vi "updateWaypoints.vi"(8 "error in (no error)":errorcluster, 11 "StationKeeping in":refnum<class "StationKeeping.lvclass">) -> (0 "error out":errorcluster, 3 "StationKeeping out":refnum<class "StationKeeping.lvclass">)   [LabVIEW 2011, in "StationKeeping.lvclass"]
doc: "Handles the 3 phases of the station keeping mission, while it is in progress. First, it checks if the mission should be started, by checking if the robot is in the station or not. If not, the start time is reset for the mission.\nIf so, using a timer, it checks which phase of the mission it is in. In the first phase, it calls \"station_keeping_waypoints.vi\" and adds waypoints to the waypoints array from a pattern in that VI. In the second phase, it adds waypoints along the edge of the boundary. These are 7 meters from the corners regardless of station size. In the third phase, it adds a waypoint outside the boundary (w/out a No-Sail Zone)\n\nThe purpose of the Local Variable \"Phase\" is to check when the phase is changing. The first time a phase changes, the \"current waypoint\" global is updated, in order to check off unecessary waypoints."
uses:
  StationKeeping.lvclass
  StationKeeping.lvclass/StationKeeping.ctl
  2 Globals/2 Global.vi
  Waypoint/Waypoint.lvclass
panel:
  out "Phase":dbl
  out "Time Elapsed":dbl
  out "Time Remaining":dbl
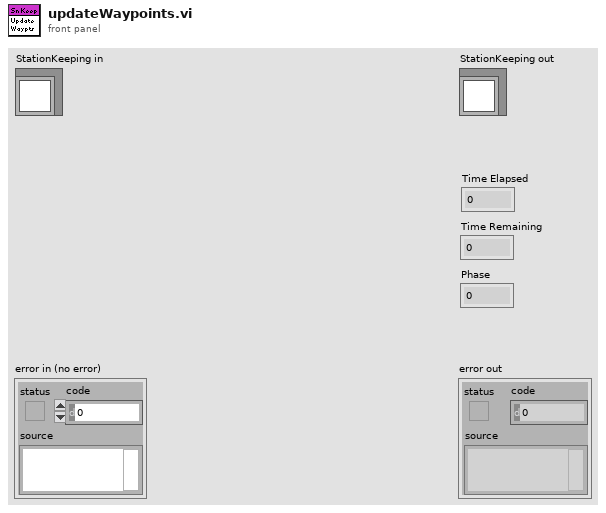
[diagram p1: front panel]
types:
  T1 = typedef "UTM Location.ctl" = cluster{"UTM Zone":dbl, "Hemisphere":enum16{"North", "South"}, "East":dbl, "North":dbl}
  T2 = typedef "UTM Circle.ctl" = cluster{"UTM Zone":dbl, "Hemisphere":enum16{"North", "South"}, "East":dbl, "North":dbl, "Radius":dbl}
  T3 = typedef "Current Waypoint.ctl" = i32
  T4 = typedef "Waypoints List.ctl" = refnum<class "Waypoint.lvclass">[]
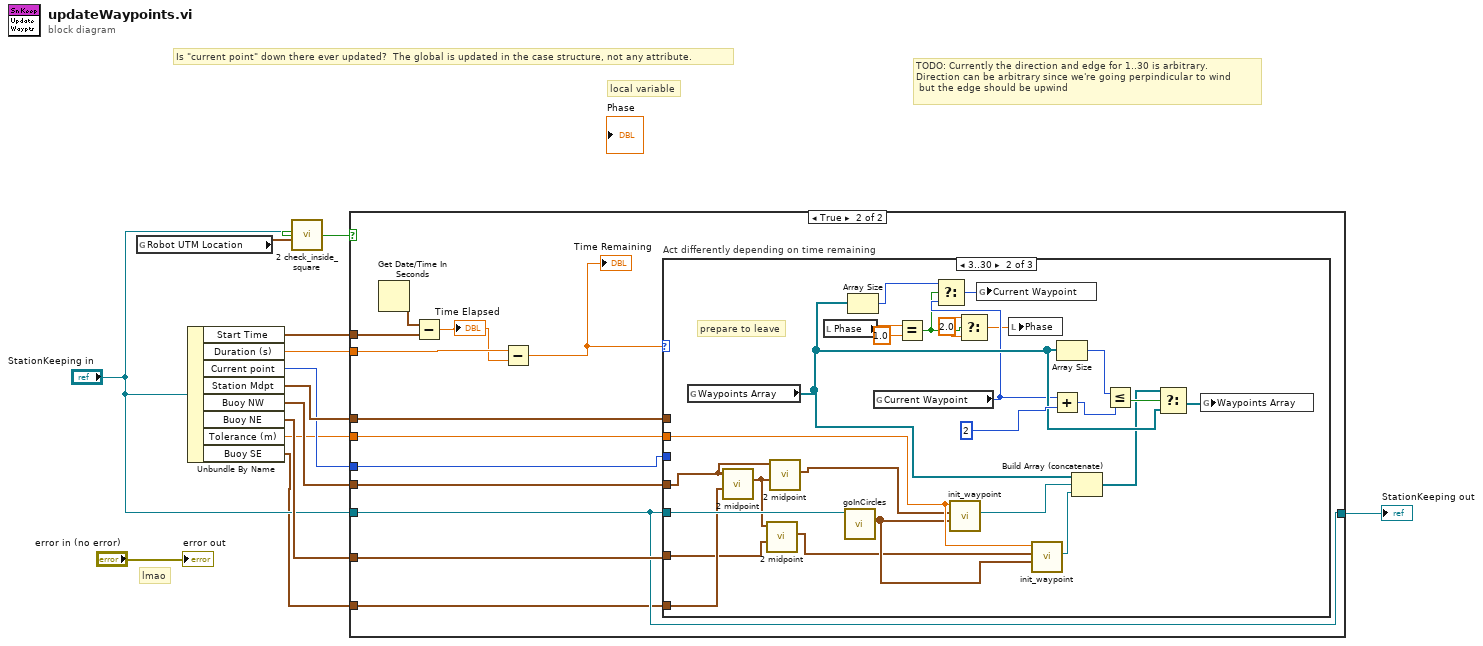
[diagram p0: block diagram]
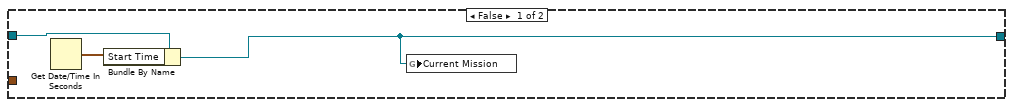
[diagram p2: hidden frame]
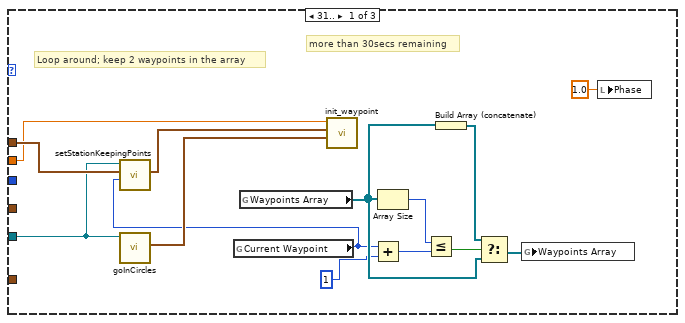
[diagram p3: hidden frame]
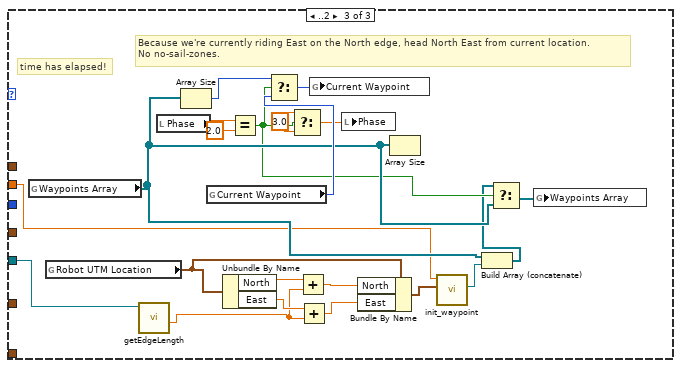
[diagram p4: hidden frame]
diagram:
  # "local variable"
  # "TODO: Currently the direction and edge for 1..30 is arbitrary.  \nDirection can be arbitrary since we're going perpindicular to wind\n but the edge should be upwind"
  # "Is \"current point\" down there ever updated?  The global is updated in the case structure, not any attribute."
  # "lmao"
  n1 = global read "2 Global.vi" "Robot UTM Location"() -> (w2:T1)
  n2 = Unbundle By Name("StationKeeping in") -> ("Start Time"=w13:timestamp, "Duration (s)"=w12:dbl, "Current point"=w7:i32, "Station Mdpt"=w11:T1, "Buoy NW"=w9:T1, "Buoy NE"=w8:T1, "Tolerance (m)"=w6:dbl, "Buoy SE"=w1:T1)
  n3 = call "2 check_inside_square.vi"("UTM Location"=w2, "StationKeeping.lvclass"="StationKeeping in") -> ("In Square?"=w4:bool)  [unwired: 9 in]
  n4 = case shown="True" w4 {
    tunnel: w13 -> [_ w27]
    tunnel: w12 -> [_ w26]
    tunnel: w11 -> [_ w24]
    tunnel: w9 -> [_ w22]
    tunnel: w8 -> [_ w21]
    tunnel: w7 -> [_ w20]
    tunnel: w6 -> [_ w19]
    tunnel: "StationKeeping in" -> [w15 w18]
    tunnel: [w14 w18] -> w5
    tunnel: w1 -> [_ w17]
    frame False {
      n5 = Get Date/Time In Seconds() -> (seconds since 1Jan1904=w16:timestamp)
      n6 = Bundle By Name(cluster=w15, "Start Time"=w16) -> (w14:refnum<class "StationKeeping.lvclass">)
      n7 = global write "2 Global.vi" "Current Mission"(w14) -> ()
    }
    frame True {
      n8 = Get Date/Time In Seconds() -> (seconds since 1Jan1904=w28:timestamp)
      n9 = Subtract(x=w28, y=w27) -> (x-y=w25:dbl)
      "Time Elapsed" <- w25
      n10 = Subtract(x=w26, y=w25) -> (x-y=w23:dbl)
      "Time Remaining" <- w23
      n11 = case "Act differently depending on time remaining" shown="3..30" w23 {
        tunnel: w20 -> [_ _ _]
        tunnel: w24 -> [w36 _ _]
        tunnel: w18 -> [w32 w49 w71]
        tunnel: w22 -> [_ w48 _]
        tunnel: w21 -> [_ w43 _]
        tunnel: w19 -> [w30 w53 w69]
        tunnel: w17 -> [_ w45 _]
        frame 31.. {
          # "more than 30secs remaining"
          # "Loop around; keep 2 waypoints in the array"
          n12 = call "goInCircles.vi"("StationKeeping in"=w32) -> ("No Sail Circles"=w35:T2[])  [unwired: 8 in, 2 out]
          n13 = global read "2 Global.vi" "Current Waypoint"() -> (w29:T3)
          n14 = call "setStationKeepingPoints.vi"("Which Point?"=w29, "Midpoint"=w36, "StationKeeping.lvclass"=w32) -> ("Waypoint"=w38:T1)  [unwired: 8 in]
          n15 = global read "2 Global.vi" "Waypoints Array"() -> (w39:T4)
          n16 = call "init_waypoint.vi"("No Sail Circles"=w35, "Coords"=w38, "Tolerance (m)"=w30) -> ()  [unwired: 8 in, 1 out]
          n17 = Add(x=w29, y=1) -> (x+y=w33:T3)
          n18 = Array Size(array=w39) -> (size(s)=w42:i32)
          n19 = Less Or Equal?(x=w42, y=w33) -> (x <= y?=w41:bool)
          n20 = Build Array (concatenate)(w39) -> (w40:T4)
          n21 = Select(t=w40, s=w41, f=w39) -> (s? t:f=w37:T4)
          n22 = global write "2 Global.vi" "Waypoints Array"(w37) -> ()
          n23 = local write "Phase"(1.0 ("Phase")) -> ()
        }
        frame 3..30 {
          w54 = 2.0 ("y")
          # "prepare to leave"
          n24 = global read "2 Global.vi" "Waypoints Array"() -> (w63:T4)
          n25 = call "2 midpoint.vi"("UTM 2"=w45, "UTM 1"=w48) -> ("Midpoint"=w46:T1)  [unwired: 8 in, 1 out]
          n26 = call "2 midpoint.vi"("UTM 2"=w43, "UTM 1"=w46) -> ("Midpoint"=w44:T1)  [unwired: 8 in, 1 out]
          n27 = call "2 midpoint.vi"("UTM 2"=w46, "UTM 1"=w48) -> ("Midpoint"=w47:T1)  [unwired: 8 in, 1 out]
          n28 = local read "Phase"() -> (w60:dbl)
          n29 = call "goInCircles.vi"("StationKeeping in"=w49) -> ("No Sail Circles"=w52:T2[])  [unwired: 8 in, 2 out]
          n30 = Array Size(array=w63) -> (size(s)=w58:i32)
          n31 = global read "2 Global.vi" "Current Waypoint"() -> (w57:T3)
          n32 = Equal?(x=w60, y=1.0) -> (x = y?=w55:bool)
          n33 = Select(t=w58, s=w55, f=w57) -> (s? t:f=w61:T3)
          n34 = call "init_waypoint.vi"("No Sail Circles"=w52, "Coords"=w47, "Tolerance (m)"=w53) -> ("Waypoint Out"=w68:refnum<class "Waypoint.lvclass">)  [unwired: 8 in]
          n35 = Select(t=w54, s=w55, f=w54) -> (s? t:f=w56:dbl)
          n36 = global write "2 Global.vi" "Current Waypoint"(w61) -> ()
          n37 = local write "Phase"(w56) -> ()
          n38 = call "init_waypoint.vi"("No Sail Circles"=w52, "Coords"=w44, "Tolerance (m)"=w53) -> ("Waypoint Out"=w67:refnum<class "Waypoint.lvclass">)  [unwired: 8 in]
          n39 = Add(x=w57, y=2) -> (x+y=w51:T3)
          n40 = Array Size(array=w63) -> (size(s)=w50:i32)
          n41 = Build Array (concatenate)(w63, w68, w67) -> (w62:T4)
          n42 = Less Or Equal?(x=w50, y=w51) -> (x <= y?=w66:bool)
          n43 = Select(t=w62, s=w66, f=w63) -> (s? t:f=w65:T4)
          n44 = global write "2 Global.vi" "Waypoints Array"(w65) -> ()
        }
        frame ..2 {
          w76 = 3.0 ("y")
          # "time has elapsed!"
          # "Because we're currently riding East on the North edge, head North East from current location.\nNo no-sail-zones."
          n45 = global read "2 Global.vi" "Waypoints Array"() -> (w75:T4)
          n46 = global read "2 Global.vi" "Robot UTM Location"() -> (w86:T1)
          n47 = call "getEdgeLength.vi"("StationKeeping in"=w71) -> ("Edge Length"=w70:dbl)  [unwired: 9 in, 1 out]
          n48 = local read "Phase"() -> (w80:dbl)
          n49 = Array Size(array=w75) -> (size(s)=w72:i32)
          n50 = global read "2 Global.vi" "Current Waypoint"() -> (w78:T3)
          n51 = Unbundle By Name(w86) -> ("North"=w88:dbl, "East"=w89:dbl)
          n52 = Equal?(x=w80, y=2.0) -> (x = y?=w74:bool)
          n53 = Select(t=w72, s=w74, f=w78) -> (s? t:f=w81:T3)
          n54 = Select(t=w76, s=w74, f=w76) -> (s? t:f=w77:dbl)
          n55 = Add(x=w88, y=w70) -> (x+y=w87:dbl)
          n56 = Add(x=w89, y=w70) -> (x+y=w85:dbl)
          n57 = global write "2 Global.vi" "Current Waypoint"(w81) -> ()
          n58 = local write "Phase"(w77) -> ()
          n59 = Bundle By Name(cluster=w86, "North"=w87, "East"=w85) -> (w83:T1)
          n60 = Array Size(array=w75) -> ()  [unwired: 1 out]
          n61 = call "init_waypoint.vi"("Coords"=w83, "Tolerance (m)"=w69) -> ("Waypoint Out"=w84:refnum<class "Waypoint.lvclass">)  [unwired: 9 in]
          n62 = Build Array (concatenate)(w75, w84) -> (w73:T4)
          n63 = Select(t=w73, s=w74, f=w75) -> (s? t:f=w82:T4)
          n64 = global write "2 Global.vi" "Waypoints Array"(w82) -> ()
        }
      }
    }
  }
  "StationKeeping out" <- w5
  "error out" <- "error in (no error)"
